vi "EdgeDetectionProcessor Create.vi"(5 "Identifier":string, 8 "error in (no error)":errorcluster, 10 "Path":path, 11 "EdgeDetectionProcessor in":refnum<class "EdgeDetectionProcessor.lvclass">) -> (0 "error out":errorcluster, 3 "EdgeDetectionProcessor out":refnum<class "EdgeDetectionProcessor.lvclass">)   [LabVIEW 2018, in "EdgeDetectionProcessor.lvclass"]
uses:
  EdgeDetectionProcessor.lvclass
  C:/Program Files/National Instruments/LabVIEW 2018/user.lib/Aaron/File IO/Video/Video Processor/Video Processor.lvclass
  <userlib>/Aaron/File IO/Video/Video Processor/Video Processor.lvclass
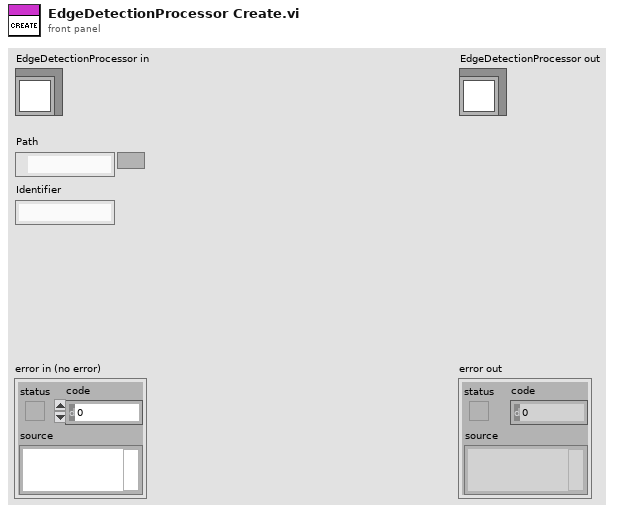
[diagram p1: front panel]
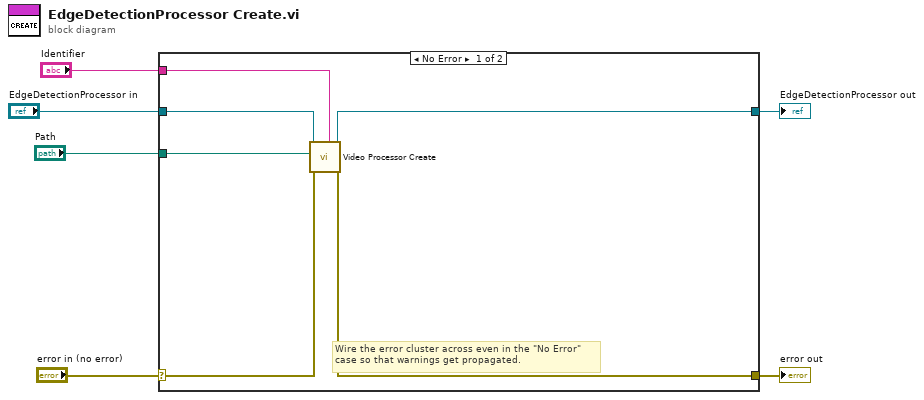
[diagram p0: block diagram]
diagram:
  n1 = case shown="No Error" "error in (no error)" {
    selector: "error in (no error)" -> [w8 w14]
    tunnel: [w7 w14] -> w5
    tunnel: [w11 w13] -> w3
    tunnel: "EdgeDetectionProcessor in" -> [w12 w13]
    tunnel: "Path" -> [w10 _]
    tunnel: "Identifier" -> [w9 _]
    frame No Error {
      # "Wire the error cluster across even in the \"No Error\"\ncase so that warnings get propagated."
      n2 = call <userlib>:"Video Processor Create.vi"("Identifier"=w9, "error in (no error)"=w8, "Video Path (\"\")"=w10, "Video Processor in"=w12) -> ("error out"=w7:errorcluster, "Video Processor out"=w11:refnum<class "EdgeDetectionProcessor.lvclass">)  [unwired: 6 in]
    }
    frame Error {
    }
  }
  "error out" <- w5
  "EdgeDetectionProcessor out" <- w3
